vi "Convert Cells into Graph.vi"(8 "error in":errorcluster, 11 "cells in":bool[][](array[boolean])) -> (0 "error out":errorcluster, 2 "game of life":T1, 3 "cells out":bool[][](array[boolean]))   [LabVIEW 2021, in "Game of Life.lvlib"]
uses:
  Game of Life.lvlib
  Graph Elements.ctl
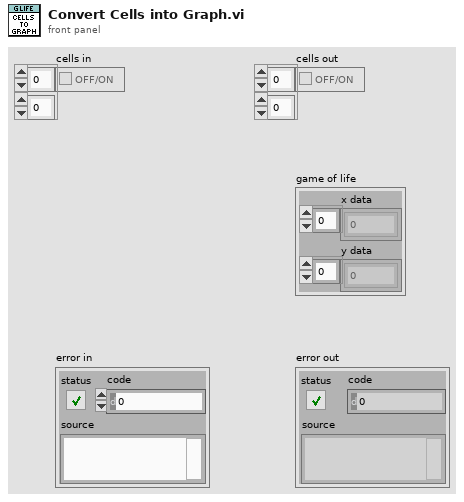
[diagram p1: front panel]
types:
  T1 = typedef "Game of Life.lvlib/Graph Elements.ctl" = cluster{"x data":dbl[], "y data":dbl[]}
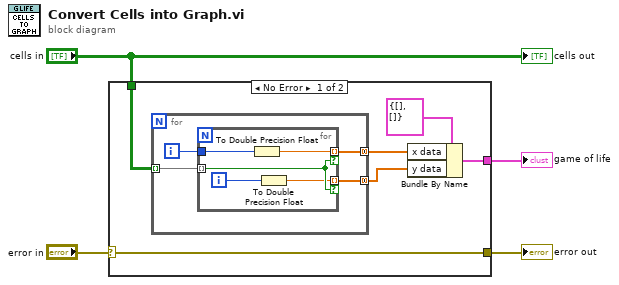
[diagram p0: block diagram]
diagram:
  n1 = case shown="No Error" "error in" {
    selector: "error in" -> [w5 w20]
    tunnel: [w9 _] -> w4
    tunnel: "cells in" -> [w6 _]
    tunnel: [w5 w20] -> w1
    frame No Error {
      n2 = for {
        tunnel: w6 -> [w14] mode=indexing
        tunnel: [w12] -> w7 mode=concatenating
        tunnel: [w11] -> w8 mode=concatenating
        i -> [w13]
        n3 = for {
          tunnel: w14 -> [w19] mode=indexing
          tunnel: [w17] -> w12 mode=indexing if=w19
          tunnel: w13 -> [w18]
          tunnel: [w15] -> w11 mode=indexing if=w19
          i -> [w16]
          n4 = To Double Precision Float(number=w18) -> (double precision float=w17:dbl)
          n5 = To Double Precision Float(number=w16) -> (double precision float=w15:dbl)
        }
      }
      n6 = Bundle By Name(cluster=T1 {"x data"=[], "y data"=[]} ("game of life"), "x data"=w7, "y data"=w8) -> (w9:T1)
    }
    frame Error {
    }
  }
  "game of life" <- w4
  "error out" <- w1
  "cells out" <- "cells in"
